vi "Get_ODE_coefficients.vi"(11 "ODE Data in":T1={"Fluid Properties"={"Fluid"=enum."Air", "Temperature (K)"=0.0, "Pressure (Pa)"=0.0}, "SJ Geometry"={"Do (mm)"=0.0, "Ho (mm)"=0.0, "Dc (mm)"=0.0, "Hc (mm)"=0.0, "Dp/Dc"=6.5}, "Solution Controls"={"Simulation"=enum."Sinusoidal", "Fixed Parameter"=enum."Pressure", "Model"=enum."Tang", "# time steps"=0, "# periods"=0, "Tolerance"=0.0, "STFT periods"=0}, "Misc Data"={"Freq jet"=1.205, "Coefficients"=[], "Nat Frequ"=1.205, "Ku"=1.205, "Scale"=1.205, "Fourier Series"=[], "Km"=1.205, "Kr"=1.205}, "Thermo and Transport Properties"={"nu"=0.0, "c"=0.0, "Pr"=0.0, "Cp"=0.0, "Cv"=0.0, "gamma"=0.0, "mu"=0.0, "rho"=0.0}, "LEM Output Data"={"X"=[], "times"=[], "|X|"=0.0, "PA X"=0.0}}) -> (3 "ODE Data out":T1={"Fluid Properties"={"Fluid"=enum."Air", "Temperature (K)"=0.0, "Pressure (Pa)"=0.0}, "SJ Geometry"={"Do (mm)"=0.0, "Ho (mm)"=0.0, "Dc (mm)"=0.0, "Hc (mm)"=0.0, "Dp/Dc"=6.5}, "Solution Controls"={"Simulation"=enum."Sinusoidal", "Fixed Parameter"=enum."Pressure", "Model"=enum."Tang", "# time steps"=0, "# periods"=0, "Tolerance"=0.0, "STFT periods"=0}, "Misc Data"={"Freq jet"=1.205, "Coefficients"=[], "Nat Frequ"=1.205, "Ku"=1.205, "Scale"=1.205, "Fourier Series"=[], "Km"=1.205, "Kr"=1.205}, "Thermo and Transport Properties"={"nu"=0.0, "c"=0.0, "Pr"=0.0, "Cp"=0.0, "Cv"=0.0, "gamma"=0.0, "mu"=0.0, "rho"=0.0}, "LEM Output Data"={"X"=[], "times"=[], "|X|"=0.0, "PA X"=0.0}})   [LabVIEW 2022 SP3]
uses:
  SJ_ODE_Data.ctl
  Utilities/fluid_properties/fluid_types.ctl
  LEM_Solution_Controls.ctl
  Model.ctl
  Fourier_Series.ctl
  Utilities/fluid_properties/fluid_properties.ctl
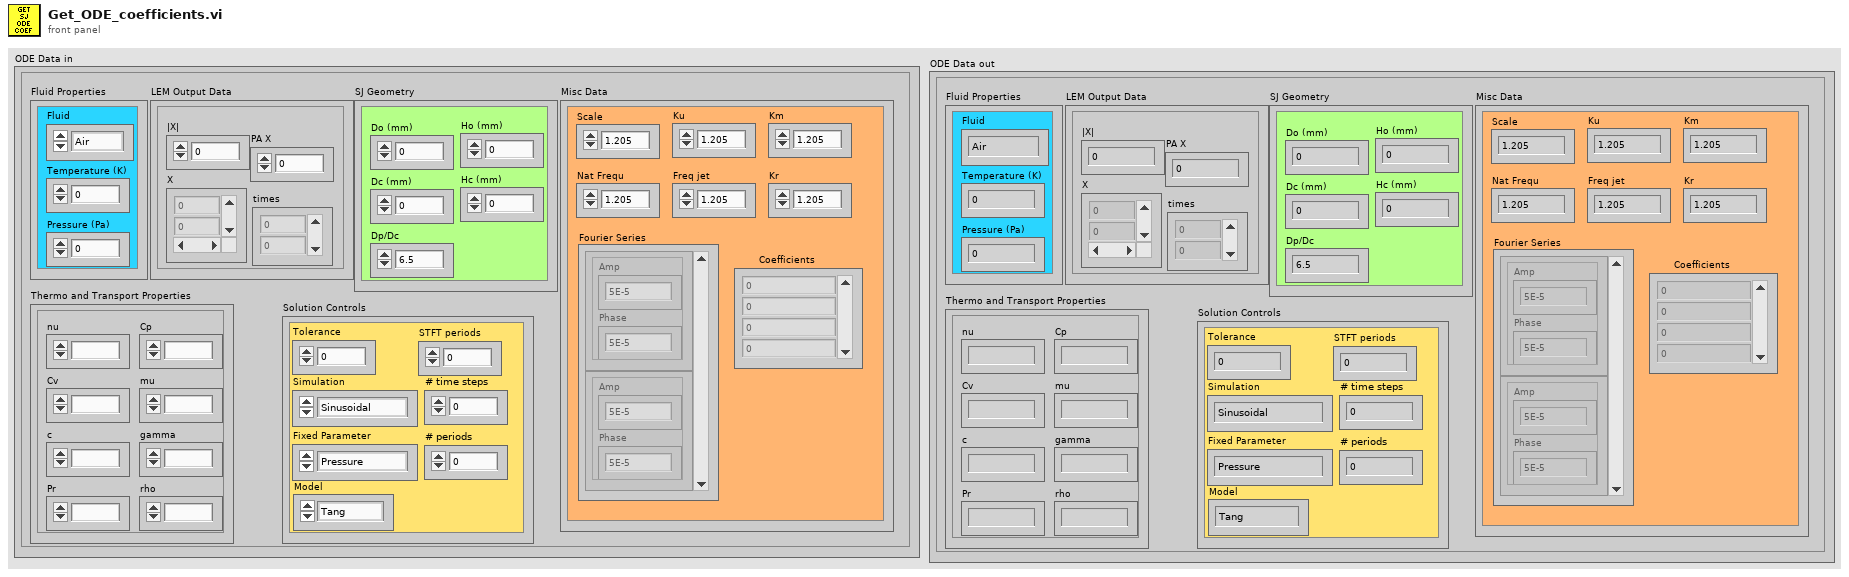
[diagram p1: front panel]
types:
  T1 = typedef "SJ_ODE_Data.ctl" = cluster{"Fluid Properties":cluster{"Fluid":T2, "Temperature (K)":dbl, "Pressure (Pa)":dbl}, "SJ Geometry":cluster{"Do (mm)":dbl, "Ho (mm)":dbl, "Dc (mm)":dbl, "Hc (mm)":dbl, "Dp/Dc":dbl}, "Solution Controls":T3, "Misc Data":cluster{"Freq jet":dbl, "Coefficients":dbl[], "Nat Frequ":dbl, "Ku":dbl, "Scale":dbl, "Fourier Series":T5, "Km":dbl, "Kr":dbl}, "Thermo and Transport Properties":T6, "LEM Output Data":cluster{"X":dbl[][], "times":dbl[], "|X|":dbl, "PA X":dbl}}
  T2 = typedef "fluid_types.ctl" = enum16{"Air", "Water"}
  T3 = typedef "LEM_Solution_Controls.ctl" = cluster{"Simulation":enum16{"Sinusoidal", "Fourier Series"}, "Fixed Parameter":enum16{"Pressure", "Displacement"}, "Model":T4, "# time steps":i32, "# periods":i32, "Tolerance":dbl, "STFT periods":i32}
  T4 = typedef "Model.ctl" = enum16{"Martin", "Tang", "Gallas", "Persoon"}
  T5 = typedef "Fourier_Series.ctl" = cluster{"Amp":dbl, "Phase":dbl}[]
  T6 = typedef "fluid_properties.ctl" = cluster{"nu":dbl, "c":dbl, "Pr":dbl, "Cp":dbl, "Cv":dbl, "gamma":dbl, "mu":dbl, "rho":dbl}
  T7 = cluster{"Fluid":T2, "Temperature (K)":dbl, "Pressure (Pa)":dbl}
  T8 = cluster{"Do (mm)":dbl, "Ho (mm)":dbl, "Dc (mm)":dbl, "Hc (mm)":dbl, "Dp/Dc":dbl}
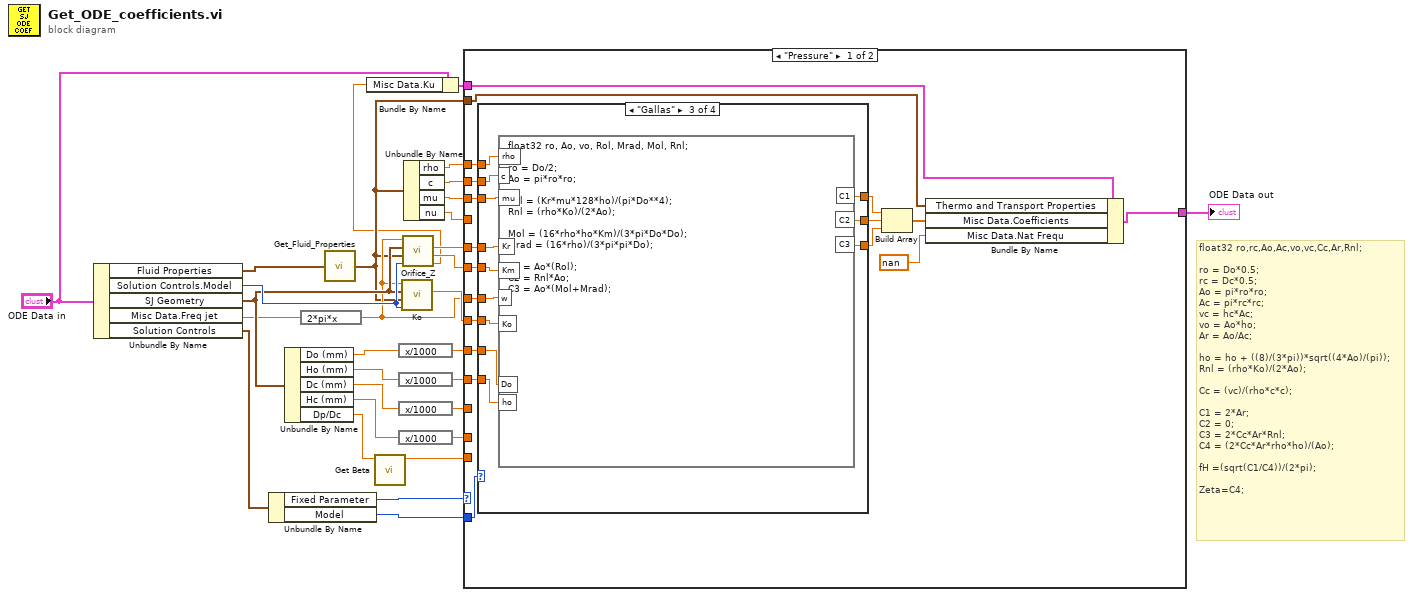
[diagram p0: block diagram]
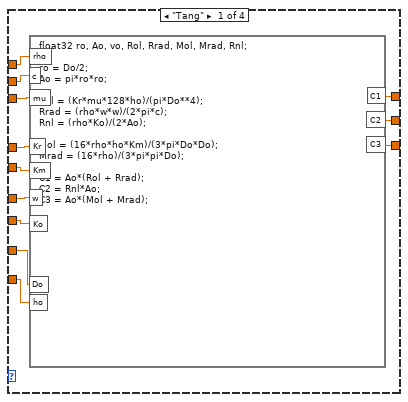
[diagram p2: hidden frame]
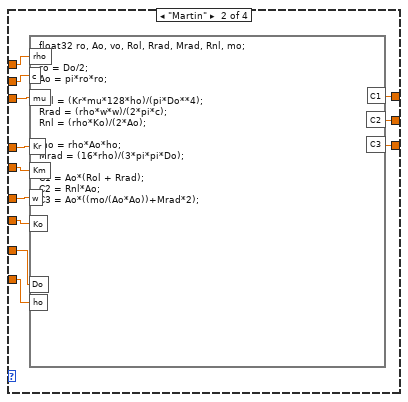
[diagram p3: hidden frame]
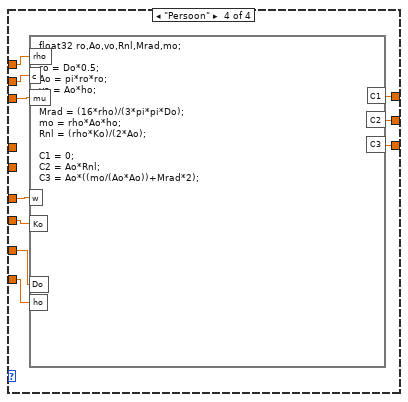
[diagram p4: hidden frame]
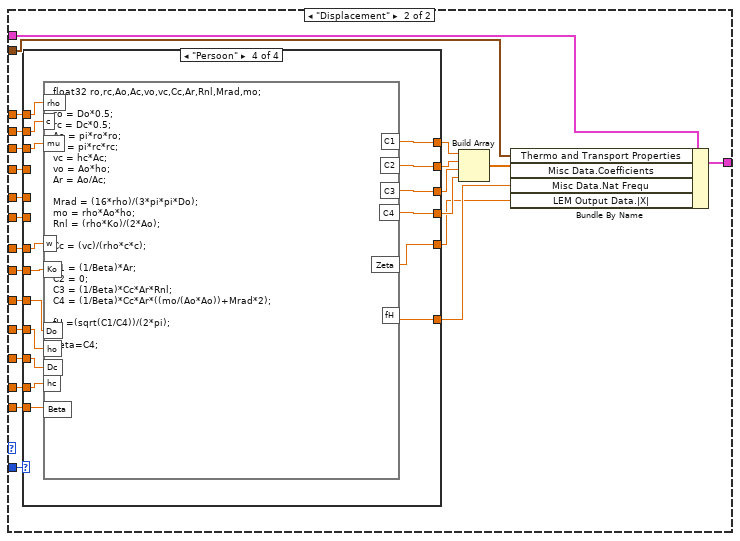
[diagram p5: hidden frame]
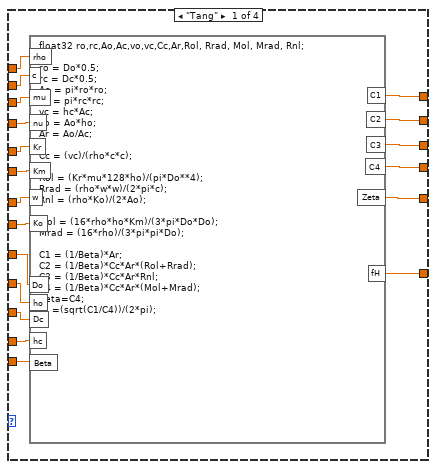
[diagram p6: hidden frame]
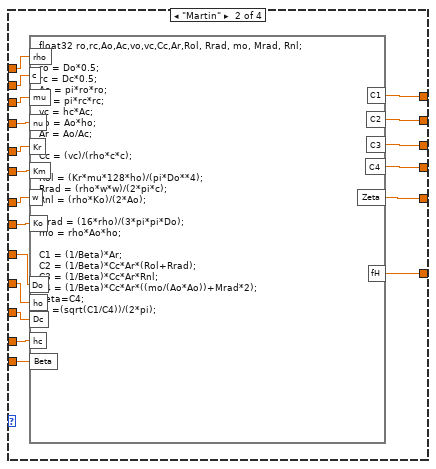
[diagram p7: hidden frame]
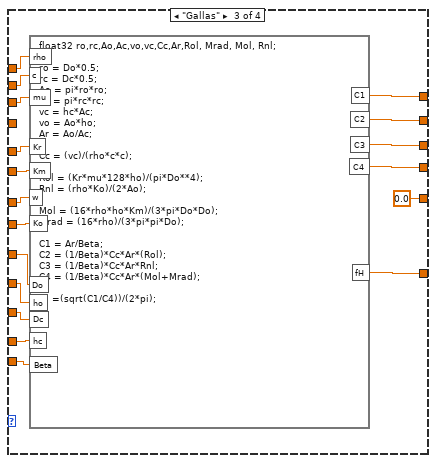
[diagram p8: hidden frame]
diagram:
  # "float32 ro,rc,Ao,Ac,vo,vc,Cc,Ar,Rnl;\n\nro = Do*0.5;\nrc = Dc*0.5;\nAo = pi*ro*ro;\nAc = pi*rc*rc;\nvc = hc*Ac;\nvo = Ao*ho; \nAr = Ao/Ac;\n\nho = ho + ((8)/(3*pi))*sqrt((4*Ao)/(pi));\nRnl = (rho*Ko)/(2*Ao);\n\nCc = (vc)/(rho*c*c);\n\nC1 = 2*Ar;\nC2 = 0;\nC3 = 2*Cc*Ar*Rnl;\nC4 = (2*Cc*Ar*rho*ho)/(Ao);\n\nfH =(sqrt(C1/C4))/(2*pi);\n\nZeta=C4;"
  n1 = Unbundle By Name("ODE Data in") -> ("Fluid Properties"=w29:T7, "Solution Controls.Model"=w30:T4, "SJ Geometry"=w24:T8, "Misc Data.Freq jet"=w8:dbl, "Solution Controls"=w28:T3)
  n2 = Unbundle By Name(w28) -> ("Fixed Parameter"=w27:enum16{"Pressure", "Displacement"}, "Model"=w26:T4)
  n3 = Unbundle By Name(w24) -> ("Do (mm)"=w23:dbl, "Ho (mm)"=w21:dbl, "Dc (mm)"=w12:dbl, "Hc (mm)"=w11:dbl, "Dp/Dc"=w2:dbl)
  n4 = expression code="2*pi*x"(w8) -> (w17:dbl)
  n5 = call "Get_Fluid_Properties.vi"("Fluid Properties"=w29) -> ("Thermo and Transport Properties"=w7:T6)  [unwired: 4 in]
  n6 = call "Get Beta.vi"("R12"=w2) -> ("Beta"=w1:dbl)  [unwired: 10 in]
  n7 = expression code="x/1000"(w23) -> (w14:dbl)
  n8 = expression code="x/1000"(w21) -> (w13:dbl)
  n9 = expression code="x/1000"(w12) -> (w10:dbl)
  n10 = expression code="x/1000"(w11) -> (w9:dbl)
  n11 = call "Ko.vi"("Model"=w30, "Thermo and Transport Properties"=w7, "SJ Geometry"=w24, "omega"=w17) -> ("Ko"=w22:dbl)  [unwired: 7 in]
  n12 = call "Orifice_Z.vi"("Model"=w30, "Thermo and Transport Properties"=w7, "SJ Geometry"=w24, "Omega"=w17) -> ("Ku"=w3:dbl, "Km"=w15:dbl, "Kr"=w16:dbl)  [unwired: 4 in, 1 out]
  n13 = Bundle By Name(cluster="ODE Data in", "Misc Data.Ku"=w3) -> (w4:T1)
  n14 = Unbundle By Name(w7) -> ("rho"=w20:dbl, "c"=w19:dbl, "mu"=w18:dbl, "nu"=w6:dbl)
  n15 = case shown="\"Pressure\"" w27 {
    tunnel: w26 -> [w48 w118]
    tunnel: w4 -> [w47 w117]
    tunnel: [w46 w116] -> w25
    tunnel: w14 -> [w41 w111]
    tunnel: w22 -> [w40 w110]
    tunnel: w13 -> [w39 w109]
    tunnel: w20 -> [w38 w108]
    tunnel: w19 -> [w37 w107]
    tunnel: w18 -> [w36 w106]
    tunnel: w17 -> [w35 w105]
    tunnel: w16 -> [w34 w104]
    tunnel: w15 -> [w33 w103]
    tunnel: w10 -> [_ w102]
    tunnel: w9 -> [_ w101]
    tunnel: w7 -> [w32 w99]
    tunnel: w6 -> [_ w96]
    tunnel: w1 -> [_ w95]
    frame "Pressure" {
      n16 = case shown="\"Gallas\"" w48 {
        tunnel: [w60 w72 w84 w94] -> w44
        tunnel: [w59 w71 w83 w93] -> w43
        tunnel: [w58 w70 w82 w92] -> w42
        tunnel: w41 -> [w57 w69 w81 w91]
        tunnel: w40 -> [w56 w68 w80 w90]
        tunnel: w39 -> [w55 w67 w79 w89]
        tunnel: w38 -> [w54 w66 w78 w88]
        tunnel: w37 -> [w53 w65 w77 w87]
        tunnel: w36 -> [w52 w64 w76 w86]
        tunnel: w35 -> [w51 w63 w75 w85]
        tunnel: w34 -> [w50 w62 w74 _]
        tunnel: w33 -> [w49 w61 w73 _]
        frame "Tang" {
          n17 = formula code="float32 ro, Ao, vo, Rol, Rrad, Mol, Mrad, Rnl;\n\nro = Do/2;\nAo = pi*ro*ro;\n\nRol = (Kr*mu*128*ho)/(pi*Do**4);\nRrad = (rho*w*w)/(2*pi*c);\nRnl = (rho*Ko)/(2*Ao);\n\nMol = (16*rho*ho*Km)/(3*pi*Do*Do);\nMrad = (16*rho)/(3*pi*pi*Do);\n\nC1 = Ao*(Rol + Rrad);\nC2 = Rnl*Ao;\nC3 = Ao*(Mol + Mrad);"("Do"=w57, "Ko"=w56, "Kr"=w50, "ho"=w55, "rho"=w54, "c"=w53, "mu"=w52, "w"=w51, "Km"=w49) -> ("C1"=w60:dbl, "C2"=w59:dbl, "C3"=w58:dbl)
        }
        frame "Martin" {
          n18 = formula code="float32 ro, Ao, vo, Rol, Rrad, Mrad, Rnl, mo;\n\nro = Do/2;\nAo = pi*ro*ro;\n\nRol = (Kr*mu*128*ho)/(pi*Do**4);\nRrad = (rho*w*w)/(2*pi*c);\nRnl = (rho*Ko)/(2*Ao);\n\nmo = rho*Ao*ho;\nMrad = (16*rho)/(3*pi*pi*Do);\n\nC1 = Ao*(Rol + Rrad);\nC2 = Rnl*Ao;\nC3 = Ao*((mo/(Ao*Ao))+Mrad*2);"("Do"=w69, "Ko"=w68, "Kr"=w62, "ho"=w67, "rho"=w66, "c"=w65, "mu"=w64, "w"=w63, "Km"=w61) -> ("C1"=w72:dbl, "C2"=w71:dbl, "C3"=w70:dbl)
        }
        frame "Gallas" {
          n19 = formula code="float32 ro, Ao, vo, Rol, Mrad, Mol, Rnl;\n\nro = Do/2;\nAo = pi*ro*ro;\n\nRol = (Kr*mu*128*ho)/(pi*Do**4);\nRnl = (rho*Ko)/(2*Ao);\n\nMol = (16*rho*ho*Km)/(3*pi*Do*Do);\nMrad = (16*rho)/(3*pi*pi*Do);\n\nC1 = Ao*(Rol);\nC2 = Rnl*Ao;\nC3 = Ao*(Mol+Mrad);"("Do"=w81, "Ko"=w80, "Kr"=w74, "ho"=w79, "rho"=w78, "c"=w77, "mu"=w76, "w"=w75, "Km"=w73) -> ("C1"=w84:dbl, "C2"=w83:dbl, "C3"=w82:dbl)
        }
        frame "Persoon" {
          n20 = formula code="float32 ro,Ao,vo,Rnl,Mrad,mo;\n\nro = Do*0.5;\nAo = pi*ro*ro;\nvo = Ao*ho; \n\nMrad = (16*rho)/(3*pi*pi*Do);\nmo = rho*Ao*ho;\nRnl = (rho*Ko)/(2*Ao);\n\nC1 = 0;\nC2 = Ao*Rnl;\nC3 = Ao*((mo/(Ao*Ao))+Mrad*2);"("Do"=w91, "Ko"=w90, "ho"=w89, "rho"=w88, "c"=w87, "mu"=w86, "w"=w85) -> ("C1"=w94:dbl, "C2"=w93:dbl, "C3"=w92:dbl)
        }
      }
      n21 = Build Array(w44, w43, w42) -> (w45:dbl[])
      n22 = Bundle By Name(cluster=w47, "Thermo and Transport Properties"=w32, "Misc Data.Coefficients"=w45, "Misc Data.Nat Frequ"=nan) -> (w46:T1)
    }
    frame "Displacement" {
      n23 = case shown="\"Persoon\"" w118 {
        tunnel: [w137 w156 w174 w190] -> w114
        tunnel: [w136 w155 w173 w189] -> w113
        tunnel: [w135 w154 w172 w188] -> w112
        tunnel: w111 -> [w134 w153 w171 w187]
        tunnel: w110 -> [w133 w152 w170 w186]
        tunnel: w109 -> [w132 w151 w169 w185]
        tunnel: w108 -> [w131 w150 w168 w184]
        tunnel: w107 -> [w130 w149 w167 w183]
        tunnel: w106 -> [w129 w148 w166 w182]
        tunnel: w105 -> [w128 w147 w165 w181]
        tunnel: w104 -> [w127 w146 w164 _]
        tunnel: w103 -> [w126 w145 w163 _]
        tunnel: w102 -> [w124 w143 w161 w179]
        tunnel: w101 -> [w123 w142 w160 w178]
        tunnel: [w125 w144 w162 w180] -> w100
        tunnel: [w122 w141 w159 w177] -> w98
        tunnel: [w121 w140 0.0 ("Zeta") w176] -> w97
        tunnel: w96 -> [w120 w139 _ _]
        tunnel: w95 -> [w119 w138 w157 w175]
        frame "Tang" {
          n24 = formula code="float32 ro,rc,Ao,Ac,vo,vc,Cc,Ar,Rol, Rrad, Mol, Mrad, Rnl;\n\nro = Do*0.5;\nrc = Dc*0.5;\nAo = pi*ro*ro;\nAc = pi*rc*rc;\nvc = hc*Ac;\nvo = Ao*ho; \nAr = Ao/Ac;\n\nCc = (vc)/(rho*c*c);\n\nRol = (Kr*mu*128*ho)/(pi*Do**4);\nRrad = (rho*w*w)/(2*pi*c);\nRnl = (rho*Ko)/(2*Ao);\n\nMol = (16*rho*ho*Km)/(3*pi*Do*Do);\nMrad = (16*rho)/(3*pi*pi*Do);\n\nC1 = (1/Beta)*Ar;\nC2 = (1/Beta)*Cc*Ar*(Rol+Rrad);\nC3 = (1/Beta)*Cc*Ar*Rnl;\nC4 = (1/Beta)*Cc*Ar*(Mol+Mrad);\nZeta=C4;\nfH =(sqrt(C1/C4))/(2*pi);"("Do"=w134, "Ko"=w133, "Kr"=w127, "ho"=w132, "rho"=w131, "c"=w130, "mu"=w129, "w"=w128, "Km"=w126, "Dc"=w124, "hc"=w123, "nu"=w120, "Beta"=w119) -> ("C1"=w137:dbl, "C2"=w136:dbl, "C3"=w135:dbl, "C4"=w125:dbl, "fH"=w122:dbl, "Zeta"=w121:dbl)
        }
        frame "Martin" {
          n25 = formula code="float32 ro,rc,Ao,Ac,vo,vc,Cc,Ar,Rol, Rrad, mo, Mrad, Rnl;\n\nro = Do*0.5;\nrc = Dc*0.5;\nAo = pi*ro*ro;\nAc = pi*rc*rc;\nvc = hc*Ac;\nvo = Ao*ho; \nAr = Ao/Ac;\n\nCc = (vc)/(rho*c*c);\n\nRol = (Kr*mu*128*ho)/(pi*Do**4);\nRrad = (rho*w*w)/(2*pi*c);\nRnl = (rho*Ko)/(2*Ao);\n\nMrad = (16*rho)/(3*pi*pi*Do);\nmo = rho*Ao*ho;\n\nC1 = (1/Beta)*Ar;\nC2 = (1/Beta)*Cc*Ar*(Rol+Rrad);\nC3 = (1/Beta)*Cc*Ar*Rnl;\nC4 = (1/Beta)*Cc*Ar*((mo/(Ao*Ao))+Mrad*2);\nZeta=C4;\nfH =(sqrt(C1/C4))/(2*pi);"("Do"=w153, "Ko"=w152, "Kr"=w146, "ho"=w151, "rho"=w150, "c"=w149, "mu"=w148, "w"=w147, "Km"=w145, "Dc"=w143, "hc"=w142, "nu"=w139, "Beta"=w138) -> ("C1"=w156:dbl, "C2"=w155:dbl, "C3"=w154:dbl, "C4"=w144:dbl, "fH"=w141:dbl, "Zeta"=w140:dbl)
        }
        frame "Gallas" {
          n26 = formula code="float32 ro,rc,Ao,Ac,vo,vc,Cc,Ar,Rol, Mrad, Mol, Rnl;\n\nro = Do*0.5;\nrc = Dc*0.5;\nAo = pi*ro*ro;\nAc = pi*rc*rc;\nvc = hc*Ac;\nvo = Ao*ho; \nAr = Ao/Ac;\n\nCc = (vc)/(rho*c*c);\n\nRol = (Kr*mu*128*ho)/(pi*Do**4);\nRnl = (rho*Ko)/(2*Ao);\n\nMol = (16*rho*ho*Km)/(3*pi*Do*Do);\nMrad = (16*rho)/(3*pi*pi*Do);\n\nC1 = Ar/Beta;\nC2 = (1/Beta)*Cc*Ar*(Rol);\nC3 = (1/Beta)*Cc*Ar*Rnl;\nC4 = (1/Beta)*Cc*Ar*(Mol+Mrad);\n\nfH =(sqrt(C1/C4))/(2*pi);"("Do"=w171, "Ko"=w170, "Kr"=w164, "ho"=w169, "rho"=w168, "c"=w167, "mu"=w166, "w"=w165, "Km"=w163, "Dc"=w161, "hc"=w160, "Beta"=w157) -> ("C1"=w174:dbl, "C2"=w173:dbl, "C3"=w172:dbl, "C4"=w162:dbl, "fH"=w159:dbl)
        }
        frame "Persoon" {
          n27 = formula code="float32 ro,rc,Ao,Ac,vo,vc,Cc,Ar,Rnl,Mrad,mo;\n\nro = Do*0.5;\nrc = Dc*0.5;\nAo = pi*ro*ro;\nAc = pi*rc*rc;\nvc = hc*Ac;\nvo = Ao*ho; \nAr = Ao/Ac;\n\nMrad = (16*rho)/(3*pi*pi*Do);\nmo = rho*Ao*ho;\nRnl = (rho*Ko)/(2*Ao);\n\nCc = (vc)/(rho*c*c);\n\nC1 = (1/Beta)*Ar;\nC2 = 0;\nC3 = (1/Beta)*Cc*Ar*Rnl;\nC4 = (1/Beta)*Cc*Ar*((mo/(Ao*Ao))+Mrad*2);\n\nfH =(sqrt(C1/C4))/(2*pi);\n\nZeta=C4;"("Do"=w187, "Ko"=w186, "ho"=w185, "rho"=w184, "c"=w183, "mu"=w182, "w"=w181, "Dc"=w179, "hc"=w178, "Beta"=w175) -> ("C1"=w190:dbl, "C2"=w189:dbl, "C3"=w188:dbl, "C4"=w180:dbl, "fH"=w177:dbl, "Zeta"=w176:dbl)
        }
      }
      n28 = Build Array(w114, w113, w112, w100) -> (w115:dbl[])
      n29 = Bundle By Name(cluster=w117, "Thermo and Transport Properties"=w99, "Misc Data.Coefficients"=w115, "Misc Data.Nat Frequ"=w98, "LEM Output Data.|X|"=w97) -> (w116:T1)
    }
  }
  "ODE Data out" <- w25
